vi "updateHeartbeat.vi"(8 "error in (no error)":errorcluster, 11 "Model in":refnum<class "Model.lvclass">) -> (0 "error out":errorcluster, 1 "resendState?":bool, 3 "Model out":refnum<class "Model.lvclass">)   [LabVIEW 2016, in "Model.lvclass"]
doc: "Publishes a return heartbeat and determines if it is appropriate to resend state information (if lost communication is restored)."
uses:
  Model.lvclass
  Typedefs/PubDataSV.ctl
  ts_sallv_exa/DataTypes/logevent_Heartbeat.ctl
  Model.lvclass/Model.ctl
  PubSubDataEvent/PubSubDataEvent.lvclass/PubSubDataEvent.ctl
  PubSubDataEvent/Read pubDataEvents.vi
  ComponentTemplateCore/ComponentModel/ComponentModel/Heartbeat/IHeartbeat/IHeartbeat.lvclass
  Typedefs/EXATypedefs.lvlib
  ts_sallv_exa/SALLV_EXA.lvlib
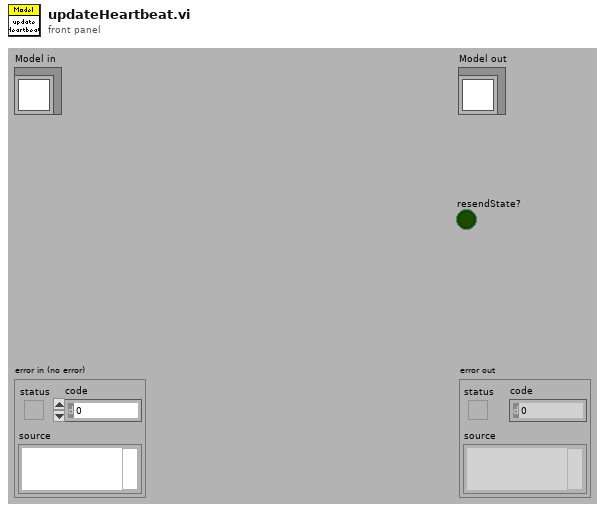
[diagram p1: front panel]
types:
  T1 = typedef "SALLV_EXA.lvlib/logevent_Heartbeat.ctl" = cluster{"heartbeat":bool, "priority":i32}
  T2 = typedef "EXATypedefs.lvlib/PubDataSV.ctl" = enum16{"DetailedState", "ErrorCode", "Heartbeat", "LoopTime_ms", "LoopTimeOutOfRange", "RejectedCommand", "SummaryState", "Timestamp", "SettingVersions", "SettingsApplied", "AppliedSettingsMatchStart"}
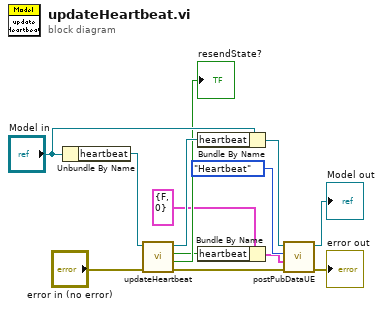
[diagram p0: block diagram]
diagram:
  n1 = Unbundle By Name("Model in") -> ("heartbeat"=w13:refnum<class "IHeartbeat.lvclass">)
  n2 = call-dynamic "updateHeartbeat.vi"("error in (no error)"="error in (no error)", "IHeartbeat in"=w13) -> ("error out"=w6:errorcluster, "resendState?"=→"resendState?":bool, "heartbeatValue"=w2:bool, "IHeartbeat out"=w10:refnum<class "IHeartbeat.lvclass">)  [unwired: 6 in]
  n3 = Bundle By Name(cluster="Model in", "heartbeat"=w10) -> (w8:refnum<class "Model.lvclass">)
  n4 = Bundle By Name(cluster=T1 {"heartbeat"=FALSE, "priority"=0} ("event data"), "heartbeat"=w2) -> (w1:T1)
  n5 = call "postPubDataUE.vi"("error in (no error)"=w6, "value"=w1, "pubDataSV"=PubDataSV."Heartbeat", "Model in"=w8) -> ("error out"=→"error out":errorcluster, "Model out"=→"Model out":refnum<class "Model.lvclass">)  [unwired: 6 in]
